vi "MDAQ_GraphCursors.vi"(9 "Status Cluster":T1 {"GATESTOP" format="%04x"; "GATESTRT" format="%04x"; "AMPLITUDE" format="%04x"; "M_CYCLES" format="%04x"; "N_CYCLES" format="%04x"; "STEP" format="%04x"; "BASE" format="%04x"; "CHAN" format="%04x"}, 10 "Input Array":u32[](array[numeric]), 11 "Graph Ref":refnum<vi>) -> (1 "Status Cluster Out":T1 {"GATESTOP" format="%04x"; "GATESTRT" format="%04x"; "AMPLITUDE" format="%04x"; "M_CYCLES" format="%04x"; "N_CYCLES" format="%04x"; "STEP" format="%04x"; "BASE" format="%04x"; "CHAN" format="%04x"}, 2 "Output Array":u32[](array[numeric]))   [LabVIEW 2021]
uses:
  Status_Cluster.ctl
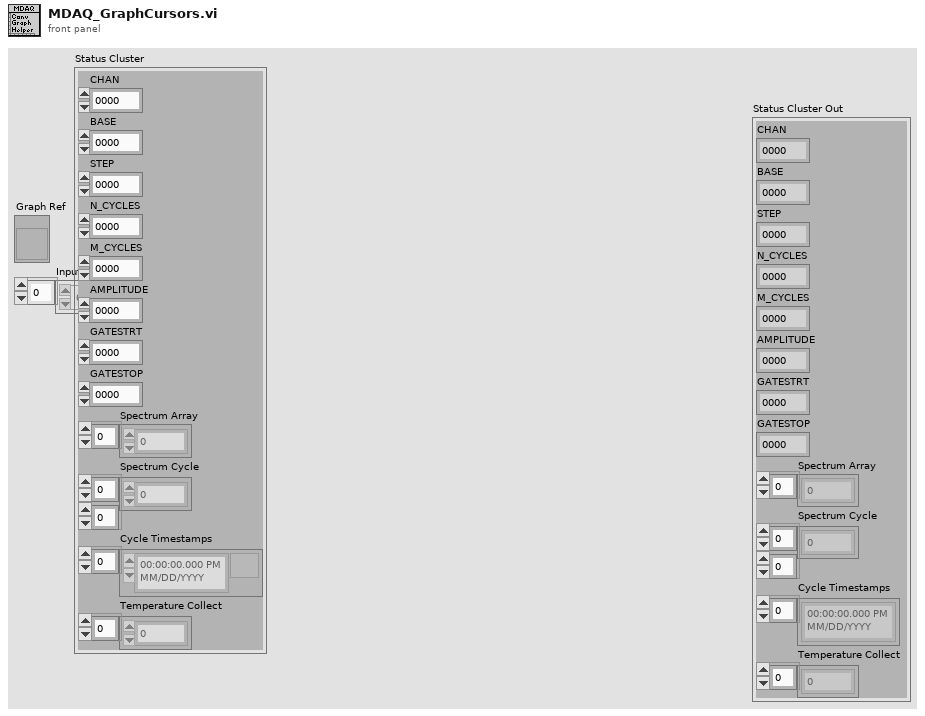
[diagram p1: front panel]
types:
  T1 = typedef "Status_Cluster.ctl" = cluster{"CHAN":u32, "BASE":u32, "STEP":u32, "N_CYCLES":u32, "M_CYCLES":u32, "AMPLITUDE":u32, "GATESTRT":u32, "GATESTOP":u32, "Spectrum Array":u32[], "Spectrum Cycle":u32[][], "Cycle Timestamps":timestamp[], "Temperature Collect":dbl[]}
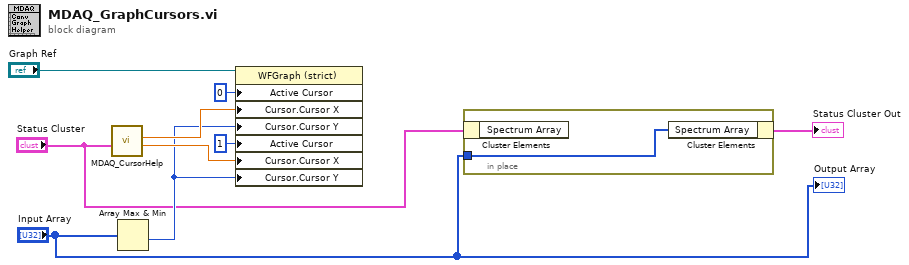
[diagram p0: block diagram]
diagram:
  n1 = call "MDAQ_CursorHelp.vi"("Input Cluster"="Status Cluster") -> ("X-Cursor-1"=w5:dbl, "X-Cursor-0"=w8:dbl)  [unwired: 9 in]
  n2 = Array Max & Min(array="Input Array") -> (min value=w4:u32)  [unwired: 3 out]
  n3 = property class="WFGraph (strict)"(reference="Graph Ref", "Active Cursor"=u32 0, "Cursor.Cursor X"=w8, "Cursor.Cursor Y"=w4, "Active Cursor"=u32 1, "Cursor.Cursor X"=w5, "Cursor.Cursor Y"=w4) -> ()  [unwired: 1 in, 2 out]
  n4 = in-place {
    in-place-border: "Input Array" -> [w10]
    n5 = in-place-cluster #1("Status Cluster") -> ()  [unwired: 1 out]
    n6 = in-place-cluster #1("Spectrum Array"=w10) -> (→"Status Cluster Out":T1)
  }
  "Output Array" <- "Input Array"
